vi "Calling_c37_118_LabVIEW_FPGA_test.vi"() -> ()   [LabVIEW 2013]
uses:
  ieeeC37_118.dll
  pmuConnectionData.dll
  <vilib>/rvi/interface/nirviReadWriteControl/nirviReadWriteControl.xnode
  <vilib>/rvi/interface/nirviOpenFPGA/nirviOpenFPGA.xnode
  <vilib>/rvi/interface/nirviCloseFPGA/nirviCloseFPGA.xnode
  FPGA Bitfiles/TestFPGA_FPGATarget_FPGA_R0cnGzbE3PM.lvbitx
  FPGA.vi
  <vilib>/FPGAPlugInAG/cRIO-9081/niLvFpga_Open_cRIO-9081.vi
  <vilib>/rvi/interface/common/dynamic/niFpgaDynamicAddResources.vi
  NiFpgaLv.dll
  <vilib>/Utility/error.llb/Error Cluster From Error Code.vi
  <vilib>/rvi/interface/Simulation/niFpgaSimulationCallBeginRW.vi
  <vilib>/rvi/errors/niLvFpgaAdjustHostInterfaceError.vi
  <vilib>/FPGAPlugInAG/Dynamic/niLvFpga_Close_Dynamic.vi
panel:
  in  "Hold Time":sgl=5000.0
  in  "alpha_POD":sgl=2.0
  in  "alpha_Load":sgl=1.81246
  in  "Scaling_Loadcontrol":sgl=120.0
  in  "Scaling_PhasorPOD":sgl=100.0
  in  "Freq of Osc POD":sgl=0.64
  in  "Freq of Osc Load":sgl=0.64
  out "Loop period monitoring 2":u8
  in  "FPGA Loop  Timer":u8=50
  out "Loop period monitoring":u32
  out "FPGA error":errorcluster
  out "Loop period RT":u8
  out "Samples\nReceived":i32
  in  "Tab Control 4":enum32{"PMUs Data Stream"}(tab)
  out "Frequency":sgl[](array[numeric])
  out "ROCOF":sgl[](array[numeric])
  out "Phasors\n(Magnitude)":sgl[](array[numeric])
  out "Phasors\n(Angle-Degree)":sgl[](array[numeric])
  out "Data Time Stamp":T1
  out "Analogs\n(Value)":sgl[](array[numeric])
  out "Phasors\n(Channel Names)":string[](array[string])
  out "Phasors\n(Types)":string[](array[string])
  out "Phasors\n(PMU Names)":string[](array[string])
  out "Analogs\n(Channel Names)":string[](array[string])
  out "Analogs\n(Types)":string[](array[string])
  out "Analogs\n(PMU Names)":string[](array[string])
  out "Data Error Status":string[](array[string])
  out "PMU Sync Status":string[](array[string])
  out "Data Processed":string[](array[string])
  out "PMU Time Quality":string[](array[string])
  out "PMU Unlocked Time":string[](array[string])
  out "PMU Triggered":string[](array[string])
  out "Trigger Reason":string[](array[string])
  in  "Tab Control 3":enum32{"Connection Data"}(tab)
  in  "IP Address (PMU / PDC)":string="130.237.53.177"
  in  "ID CODE":i32=787
  in  "Port Number":i32=38068
  in  "Tab Control 2":enum32{"PMUs Configuration"}(tab)
  out "Number of\nAnalogs":u16[](array[numeric])
  out "Number of\nDigitals":u16[](array[numeric])
  out "Nominal\nFrequency":sgl[](array[numeric])
  out "Configuration\nCount":u16[](array[numeric])
  out "Number of\nPhasors":u16[](array[numeric])
  out "Station\nName":string[](array[string])
  out "ID Code":u16[](array[numeric])
  in  "Tab Control":enum32{"PDC Configuration"}(tab)
  out "Data Rate:":u16
  out "Number of PMUs:":u16
  out "Configuration Time Stamp":T2
  in  "Shut Down":bool
  out "Error with dll client":errorcluster
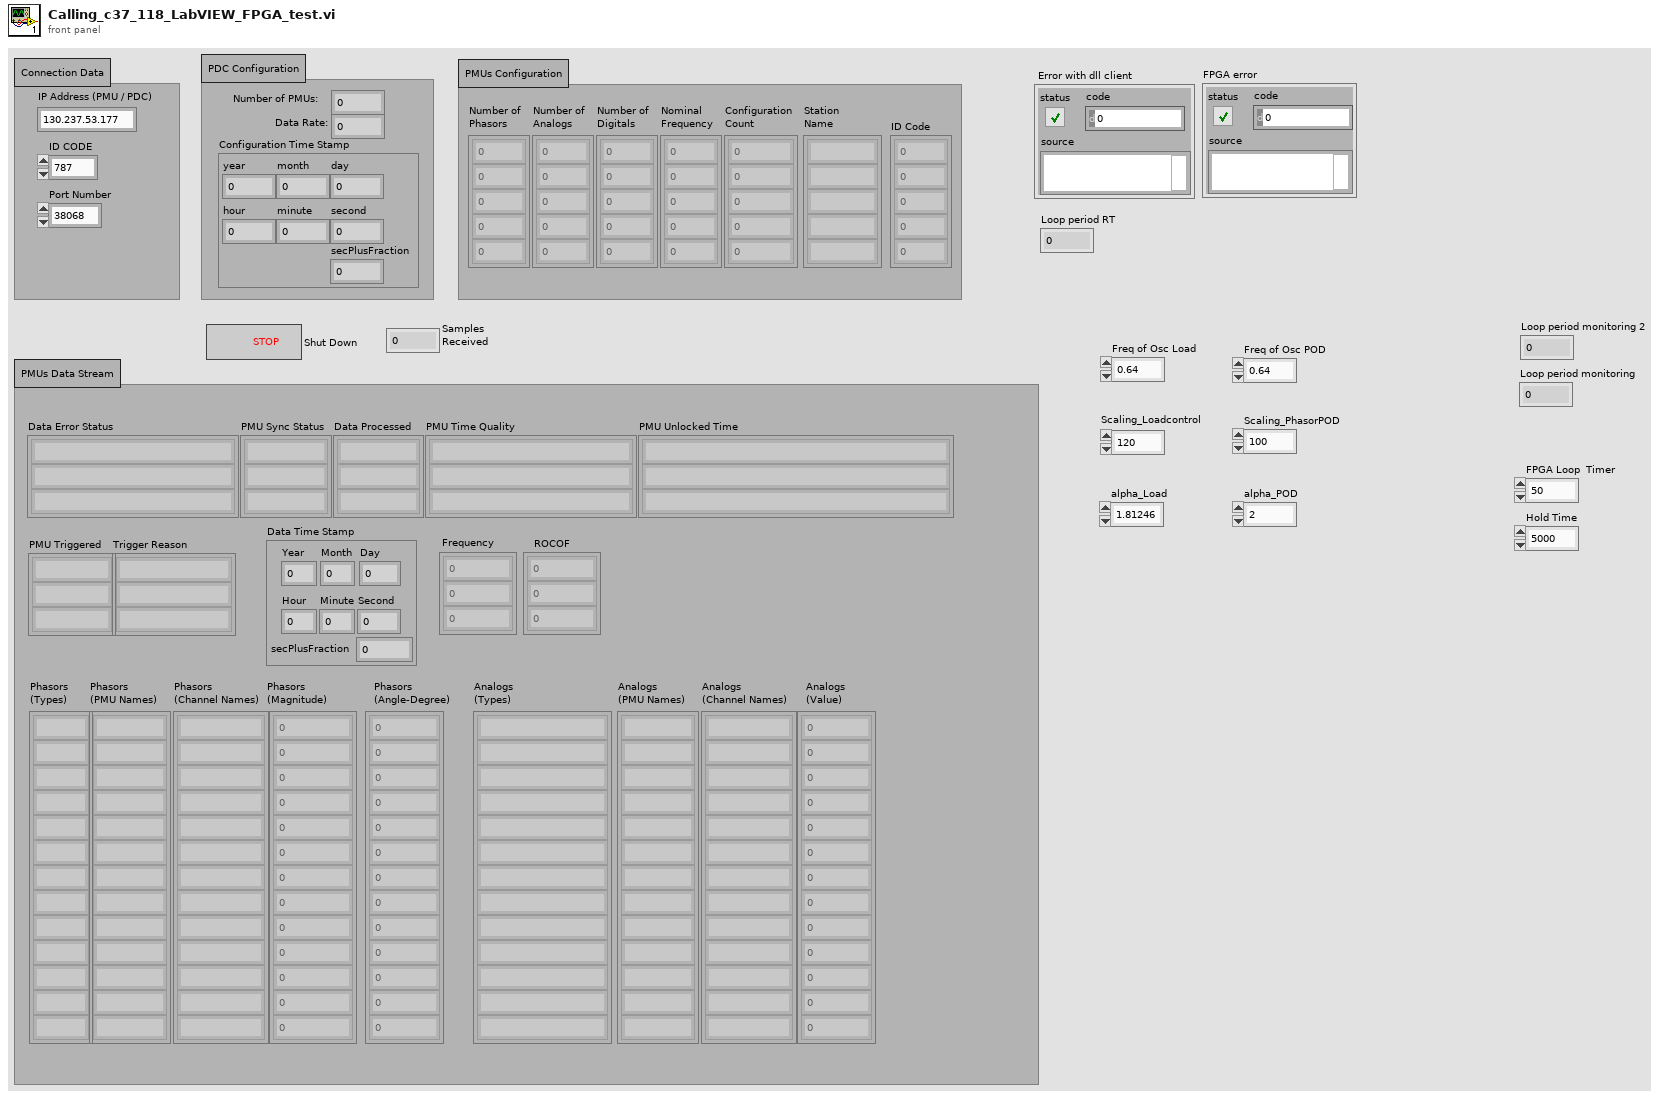
[diagram p1: front panel]
types:
  T1 = cluster{"Year":i32, "Month":i32, "Day":i32, "Hour":i32, "Minute":i32, "Second":i32, "secPlusFraction":sgl}
  T2 = cluster{"year":i32, "month":i32, "day":i32, "hour":i32, "minute":i32, "second":i32, "secPlusFraction":sgl}
  T3 = cluster{"dataError":u8, "dataModified":u8, "pmuIsNOTSync":u8, "pmuIsTriggered":u8, "pmuTimeQuality":u8, "triggerReason":u8, "unlockTime":u8}
  T4 = cluster{"Parameters":cluster{"Ts":sgl, "kappaav":sgl, "kappaph":sgl, "mu":sgl}}
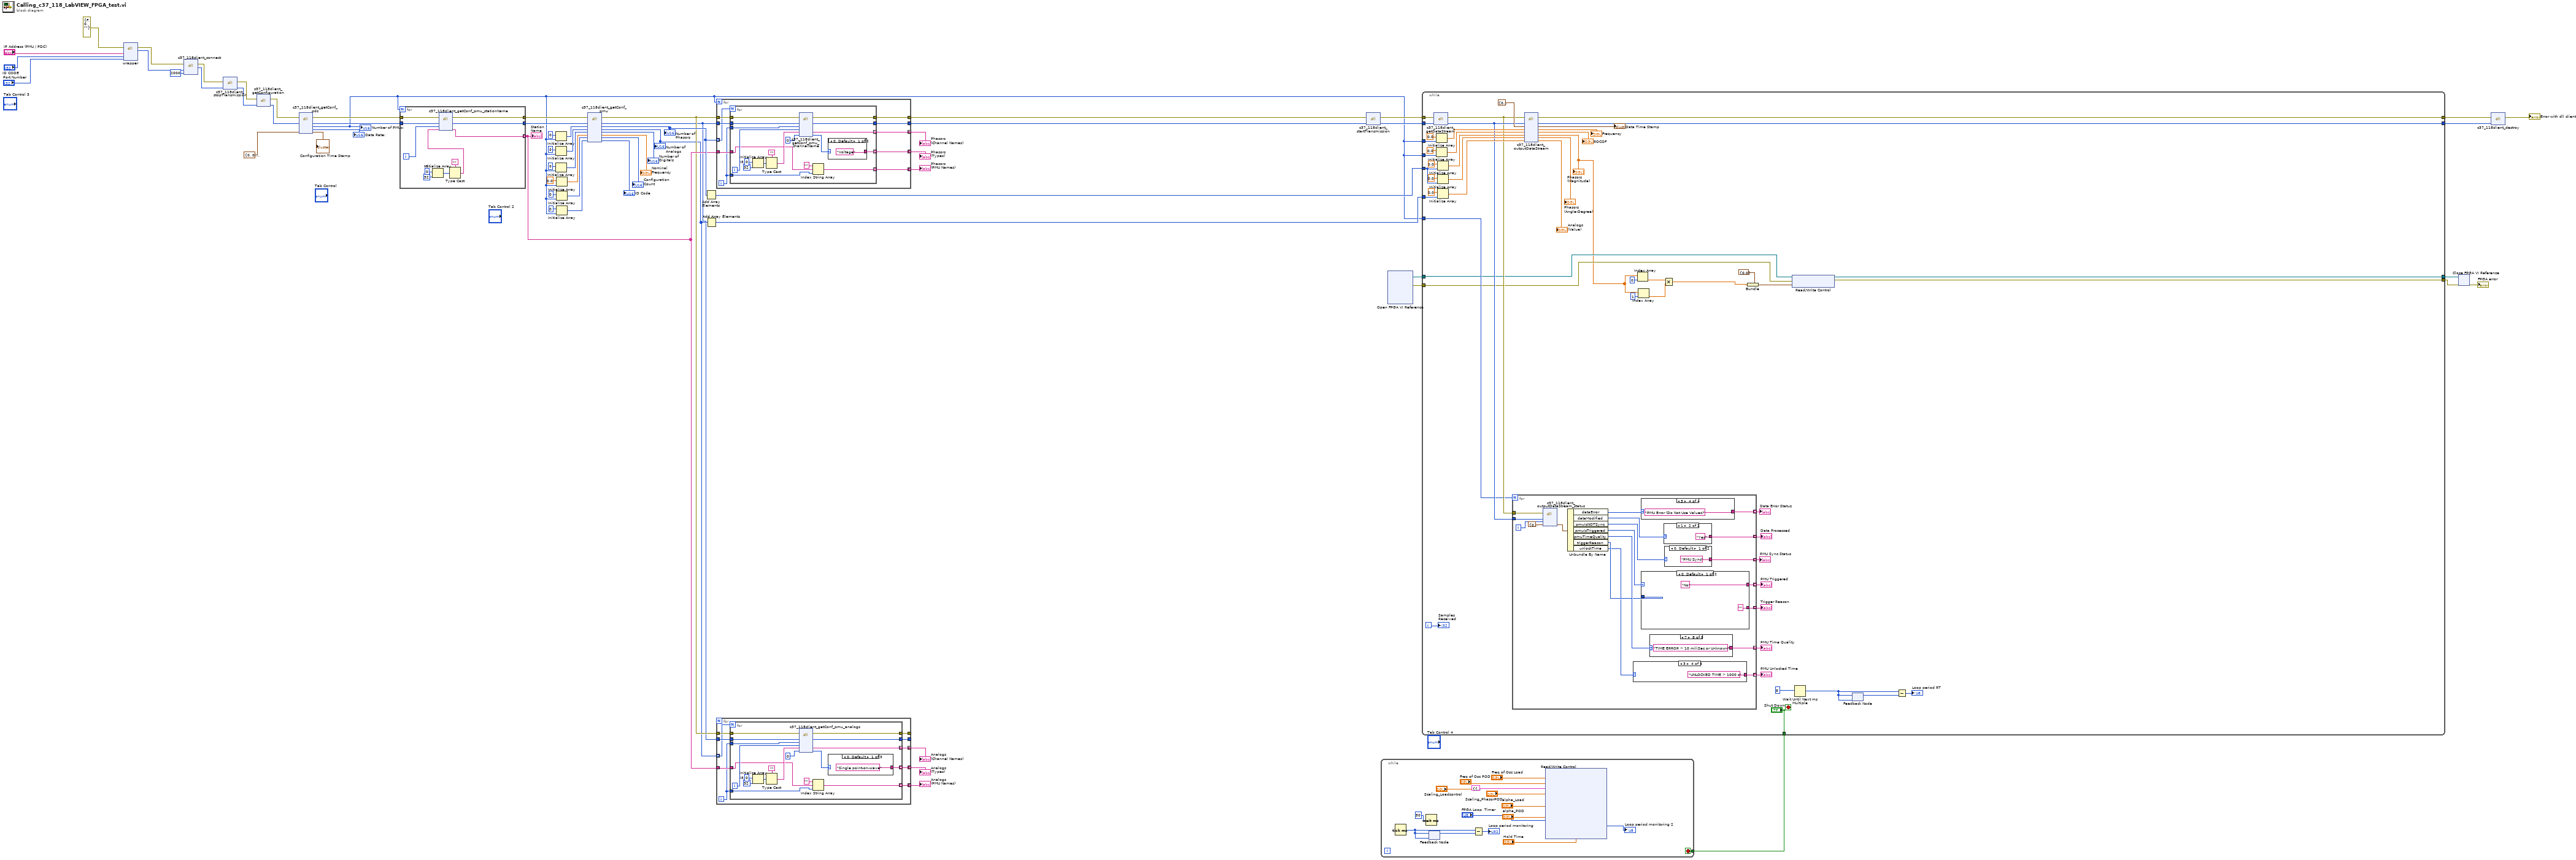
[diagram p0: block diagram]
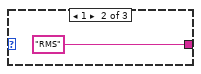
[diagram p2: hidden frame]
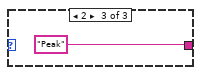
[diagram p3: hidden frame]
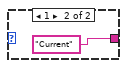
[diagram p4: hidden frame]
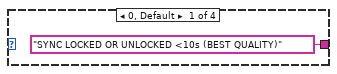
[diagram p5: hidden frame]
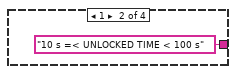
[diagram p6: hidden frame]
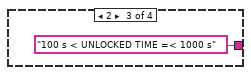
[diagram p7: hidden frame]
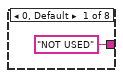
[diagram p8: hidden frame]
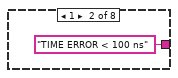
[diagram p9: hidden frame]
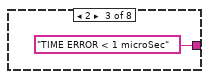
[diagram p10: hidden frame]
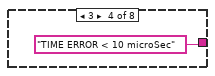
[diagram p11: hidden frame]
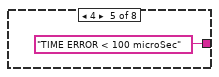
[diagram p12: hidden frame]
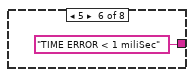
[diagram p13: hidden frame]
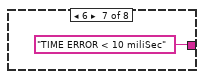
[diagram p14: hidden frame]
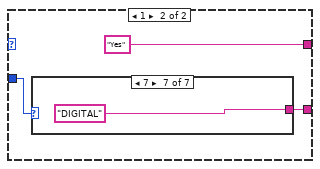
[diagram p15: hidden frame]
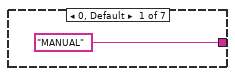
[diagram p16: hidden frame]
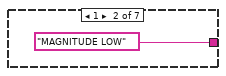
[diagram p17: hidden frame]
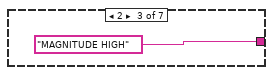
[diagram p18: hidden frame]
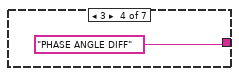
[diagram p19: hidden frame]
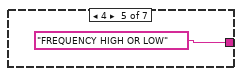
[diagram p20: hidden frame]
diagram:
  n1 = dll-call lib="pmuConnectionData.*" fn="wrapper"(error in=errorcluster {"status"=FALSE, "code"=0, "source"=""} ("error in (no error)"), "ipAddress_PmuServer"="IP Address (PMU / PDC)", "pmuPortNumber"="ID CODE", "pmuIdCode"="Port Number") -> (error out=w54:errorcluster, "PMUConnectionData"=w63:i64)  [unwired: 5 in, 1 out]
  n2 = dll-call lib="ieeeC37_118.*" fn="c37_118client_connect"(error in=w54, "parameters"=w63, "timeoutInMs"=u32 2000) -> (error out=w53:errorcluster, "c37_118Object"=w61:i64)  [unwired: 4 in, 1 out]
  n3 = dll-call lib="ieeeC37_118.dll" fn="c37_118client_stopTransmission"(error in=w53, "self"=w61) -> (error out=w52:errorcluster, "self"=w60:i64)  [unwired: 3 in, 1 out]
  n4 = dll-call lib="ieeeC37_118.dll" fn="c37_118client_getConfiguration"(error in=w52, "self"=w60) -> (error out=w51:errorcluster, "self"=w57:i64)  [unwired: 3 in, 1 out]
  n5 = dll-call lib="ieeeC37_118.dll" fn="c37_118client_getConf_pdc"(error in=w51, "self"=w57, "timestamp"=T2 {"year"=0, "month"=0, "day"=0, "hour"=0, "minute"=0, "second"=0, "secPlusFraction"=0.0}) -> (error out=w28:errorcluster, "self"=w26:i64, "num_pmu"=w7:u16, "data_rate"=→"Data Rate:":u16, "timestamp"=→"Configuration Time Stamp":T2)  [unwired: 5 in, 1 out]
  "Number of PMUs:" <- w7
  n6 = for {
    N: w7 -> [_]
    tunnel: w28 -> [w74]
    tunnel: [w73] -> w27
    tunnel: w26 -> [w72]
    tunnel: [w71] -> w25
    tunnel: [w70] -> w11 mode=indexing
    i -> [w64]
    w69 = i8 0  # I8
    n7 = Initialize Array(w69, 32 ("dimension size")) -> (w68:i8[])
    n8 = Type Cast(type="", x=w68) -> (*(type *) &x=w66:string)
    n9 = dll-call lib="ieeeC37_118.dll" fn="c37_118client_getConf_pmu_stationName"(error in=w74, "self"=w72, "pmuNumber"=w64, "stationName"=w66) -> (error out=w73:errorcluster, "self"=w71:i64, "stationName"=w70:string)  [unwired: 4 in, 1 out]
  }
  "Station\nName" <- w11
  n10 = Initialize Array(u16 0 ("element"), w7) -> (w44:u16[])
  n11 = Initialize Array(u16 0 ("element"), w7) -> (w41:u16[])
  n12 = Initialize Array(u16 0 ("element"), w7) -> (w37:u16[])
  n13 = Initialize Array(sgl 0.0 ("element"), w7) -> (w36:sgl[])
  n14 = Initialize Array(u16 0 ("element"), w7) -> (w35:u16[])
  n15 = Initialize Array(u16 0 ("element"), w7) -> (w18:u16[])
  n16 = dll-call lib="ieeeC37_118.dll" fn="c37_118client_getConf_pmu"(error in=w27, "self"=w25, "numPhasors"=w44, "numAnalog"=w41, "numdigital"=w37, "freqNom"=w36, "configCount"=w35, "idCode"=w18) -> (error out=w10:errorcluster, "self"=w8:i64, "numPhasors"=w22:u16[], "numAnalog"=w9:u16[], "numdigital"=→"Number of\nDigitals":u16[], "freqNom"=→"Nominal\nFrequency":sgl[], "configCount"=→"Configuration\nCount":u16[], "idCode"=→"ID Code":u16[])  [unwired: 3 in, 1 out]
  "Number of\nAnalogs" <- w9
  "Number of\nPhasors" <- w22
  n17 = Add Array Elements(numeric array=w22) -> (sum=w24:u16)
  n18 = Add Array Elements(numeric array=w9) -> (sum=w29:u16)
  n19 = for {
    N: w7 -> [_]
    tunnel: w10 -> [w83]
    tunnel: [w82] -> w12
    tunnel: w8 -> [w84]
    tunnel: [w81] -> w13
    tunnel: [w80] -> w23 mode=concatenating
    tunnel: w22 -> [w79] mode=indexing
    tunnel: [w78] -> w21 mode=concatenating
    tunnel: w11 -> [w77]
    tunnel: [w75] -> w20 mode=concatenating
    i -> [w76]
    n20 = for {
      N: w79 -> [_]
      tunnel: w76 -> [w97]
      tunnel: w84 -> [w96]
      tunnel: w83 -> [w95]
      tunnel: [w94] -> w82
      tunnel: [w93] -> w81
      tunnel: [w92] -> w80 mode=indexing
      tunnel: [w89] -> w78 mode=indexing
      tunnel: w77 -> [w87]
      tunnel: w76 -> [w88]
      tunnel: [w85] -> w75 mode=indexing
      i -> [w98]
      w103 = i8 0  # I8
      n21 = Initialize Array(w103, 32 ("dimension size")) -> (w102:i8[])
      n22 = Type Cast(type="", x=w102) -> (*(type *) &x=w99:string)
      n23 = dll-call lib="ieeeC37_118.dll" fn="c37_118client_getConf_pmu_channelName"(error in=w95, "self"=w96, "pmuNumber"=w97, "phasor"=w98, "channelName"=w99, "phasorType"=0) -> (error out=w94:errorcluster, "self"=w93:i64, "channelName"=w92:string, "phasorType"=w90:i32)  [unwired: 5 in, 1 out]
      n24 = Index String Array(1:w88, 2:w87, 3:"" ("string (\"\")")) -> (0:w85:string)
      n25 = case shown="0, Default" w90 {
        tunnel: ["Voltage" "Current"] -> w89
        frame 0, Default {
        }
        frame 1 {
        }
      }
    }
  }
  "Phasors\n(Channel Names)" <- w23
  "Phasors\n(Types)" <- w21
  "Phasors\n(PMU Names)" <- w20
  n26 = for {
    tunnel: w10 -> [w114]
    tunnel: [w113] -> _
    tunnel: w8 -> [w115]
    tunnel: [w112] -> _
    tunnel: [w111] -> w16 mode=concatenating
    tunnel: w9 -> [w110] mode=indexing
    tunnel: [w109] -> w15 mode=concatenating
    tunnel: w11 -> [w108]
    tunnel: [w106] -> w14 mode=concatenating
    i -> [w107]
    n27 = for {
      N: w110 -> [_]
      tunnel: w107 -> [w128]
      tunnel: w115 -> [w127]
      tunnel: w114 -> [w126]
      tunnel: [w125] -> w113
      tunnel: [w124] -> w112
      tunnel: [w123] -> w111 mode=indexing
      tunnel: [w120] -> w109 mode=indexing
      tunnel: w108 -> [w118]
      tunnel: w107 -> [w119]
      tunnel: [w116] -> w106 mode=indexing
      i -> [w129]
      w134 = i8 0  # I8
      n28 = Initialize Array(w134, 32 ("dimension size")) -> (w133:i8[])
      n29 = Type Cast(type="", x=w133) -> (*(type *) &x=w130:string)
      n30 = dll-call lib="ieeeC37_118.dll" fn="c37_118client_getConf_pmu_analogs"(error in=w126, "self"=w127, "pmuNumber"=w128, "analog"=w129, "channelName"=w130, "analogType"=0 ("phasorType")) -> (error out=w125:errorcluster, "self"=w124:i64, "channelName"=w123:string, "analogType"=w121:i32)  [unwired: 5 in, 1 out]
      n31 = Index String Array(1:w119, 2:w118, 3:"" ("string (\"\")")) -> (0:w116:string)
      n32 = case shown="0, Default" w121 {
        tunnel: ["Single point-on-wave" "RMS" "Peak"] -> w120
        frame 0, Default {
        }
        frame 1 {
        }
        frame 2 {
        }
      }
    }
  }
  "Analogs\n(Channel Names)" <- w16
  "Analogs\n(Types)" <- w15
  "Analogs\n(PMU Names)" <- w14
  n33 = dll-call lib="ieeeC37_118.dll" fn="c37_118client_startTransmission"(error in=w12, "self"=w13) -> (error out=w50:errorcluster, "self"=w59:i64)  [unwired: 3 in, 1 out]
  n34 = xnode "Open FPGA VI Reference"() -> ("FPGA VI Reference Out"=w6:refnum<k20>, "error out"=w5:errorcluster)  [unwired: 2 in]
  n35 = while {
    tunnel: w59 -> [w189]
    tunnel: [w186] -> w58
    tunnel: w50 -> [w188]
    tunnel: [w187] -> w49
    tunnel: w7 -> [w184]
    tunnel: w7 -> [w181]
    tunnel: w24 -> [w175]
    tunnel: w29 -> [w168]
    tunnel: w7 -> [w164]
    tunnel: w6 -> [w149]
    tunnel: w5 -> [w150]
    tunnel: [w148] -> w4
    tunnel: [w147] -> w3
    tunnel: ["Shut Down"] -> w1
    i -> [w170]
    stop <- "Shut Down" stop-if-true
    n36 = dll-call lib="ieeeC37_118.dll" fn="c37_118client_getDataStream"(error in=w188, "self"=w189) -> (error out=w165:errorcluster, "self"=w166:i64)  [unwired: 3 in, 1 out]
    n37 = Initialize Array(sgl 0.0 ("element"), w184) -> (w183:sgl[])
    n38 = Initialize Array(sgl 0.0 ("element"), w181) -> (w180:sgl[])
    n39 = Initialize Array(sgl 0.0 ("element"), w175) -> (w174:sgl[])
    n40 = Initialize Array(sgl 0.0 ("element"), w175) -> (w173:sgl[])
    n41 = Initialize Array(sgl 0.0 ("element"), w168) -> (w167:sgl[])
    n42 = for {
      N: w164 -> [_]
      tunnel: w166 -> [w208]
      tunnel: w165 -> [w207]
      tunnel: [w204] -> w163 mode=indexing
      tunnel: [w201] -> w162 mode=indexing
      tunnel: [w198] -> w161 mode=indexing
      tunnel: [w196] -> w160 mode=indexing
      tunnel: [w195] -> w159 mode=indexing
      tunnel: [w192] -> w158 mode=indexing
      tunnel: [w190] -> w157 mode=indexing
      i -> [w206]
      n43 = dll-call lib="ieeeC37_118.dll" fn="c37_118client_outputDataStream_status"(error in=w207, "self"=w208, "pmuNumber"=w206, "status"=T3 {"dataError"=0, "dataModified"=0, "pmuIsNOTSync"=0, "pmuIsTriggered"=0, "pmuTimeQuality"=0, "triggerReason"=0, "unlockTime"=0}) -> ("status"=w203:T3)  [unwired: 5 in, 2 out]
      n44 = Unbundle By Name(w203) -> ("dataError"=w200:u8, "dataModified"=w199:u8, "pmuIsNOTSync"=w202:u8, "pmuIsTriggered"=w197:u8, "pmuTimeQuality"=w194:u8, "triggerReason"=w193:u8, "unlockTime"=w191:u8)
      n45 = case shown="3" w191 {
        tunnel: ["SYNC LOCKED OR UNLOCKED <10s (BEST QUALITY)" "10 s =< UNLOCKED TIME < 100 s" "100 s < UNLOCKED TIME =< 1000 s" "UNLOCKED TIME > 1000 s"] -> w190
        frame 0, Default {
        }
        frame 1 {
        }
        frame 2 {
        }
        frame 3 {
        }
      }
      n46 = case shown="3" w200 {
        tunnel: ["Good Measurment Data (No Errors)" "PMU Error, No Information About Data" "PMU In Test Mode (Do Not Use Values)" "PMU Error (Do Not Use Values)"] -> w204
        frame 0, Default {
        }
        frame 1 {
        }
        frame 2 {
        }
        frame 3 {
        }
      }
      n47 = case shown="0, Default" w197 {
        tunnel: ["No" "Yes"] -> w196
        tunnel: w193 -> [_ w224]
        tunnel: ["" w223] -> w192
        frame 0, Default {
        }
        frame 1 {
          n48 = case shown="7" w224 {
            tunnel: ["MANUAL" "MAGNITUDE LOW" "MAGNITUDE HIGH" "PHASE ANGLE DIFF" "FREQUENCY HIGH OR LOW" "df/dt HIGH" "DIGITAL"] -> w223
            frame 0, Default {
            }
            frame 1 {
            }
            frame 2 {
            }
            frame 3 {
            }
            frame 4 {
            }
            frame 5 {
            }
            frame 7 {
            }
          }
        }
      }
      n49 = case shown="7" w194 {
        tunnel: ["NOT USED" "TIME ERROR < 100 ns" "TIME ERROR < 1 microSec" "TIME ERROR < 10 microSec" "TIME ERROR < 100 microSec" "TIME ERROR < 1 miliSec" "TIME ERROR < 10 miliSec" "TIME ERROR > 10 miliSec or Unknown"] -> w195
        frame 0, Default {
        }
        frame 1 {
        }
        frame 2 {
        }
        frame 3 {
        }
        frame 4 {
        }
        frame 5 {
        }
        frame 6 {
        }
        frame 7 {
        }
      }
      n50 = case shown="1" w199 {
        tunnel: ["No" "Yes"] -> w198
        frame 0, Default {
        }
        frame 1 {
        }
      }
      n51 = case shown="0, Default" w202 {
        tunnel: ["PMU Sync" "PMU Not Sync"] -> w201
        frame 0, Default {
        }
        frame 1 {
        }
      }
    }
    "Data Error Status" <- w163
    "PMU Sync Status" <- w162
    "Data Processed" <- w161
    "PMU Triggered" <- w160
    "PMU Time Quality" <- w159
    "Trigger Reason" <- w158
    "PMU Unlocked Time" <- w157
    n52 = dll-call lib="ieeeC37_118.dll" fn="c37_118client_outputDataStream"(error in=w165, "self"=w166, "timestamp"=T2 {"year"=0, "month"=0, "day"=0, "hour"=0, "minute"=0, "second"=0, "secPlusFraction"=0.0}, "freqBuffer"=w183, "rocofBuffer"=w180, "phasorsMagBuffer"=w174, "phasorsAngBuffer"=w173, "analogBuffer"=w167) -> (error out=w187:errorcluster, "self"=w186:i64, "timestamp"=→"Data Time Stamp":T2, "freqBuffer"=→"Frequency":sgl[], "rocofBuffer"=→"ROCOF":sgl[], "phasorsMagBuffer"=w139:sgl[], "phasorsAngBuffer"=→"Phasors\n(Angle-Degree)":sgl[], "analogBuffer"=→"Analogs\n(Value)":sgl[])  [unwired: 3 in, 1 out]
    "Phasors\n(Magnitude)" <- w139
    n53 = Index Array(array=w139, index=0) -> (element=w143:sgl)
    n54 = Index Array(array=w139, index=1) -> (element=w142:sgl)
    n55 = Multiply(x=w143, y=w142) -> (x*y=w141:sgl)
    n56 = Bundle(cluster=cluster{sgl} {0.0}, w141) -> (w146:cluster{sgl})
    n57 = xnode "Read/Write Control"("FPGA VI Reference In"=w149, "error in"=w150, "PMU measurments"=w146) -> ("FPGA VI Reference Out"=w148:refnum<k20>, "error out"=w147:errorcluster)
    n58 = Wait Until Next ms Multiple(millisecond multiple=u32 5) -> (millisecond timer value=w152:u32)
    n59 = feedback #1(w152) -> (w154:u32)
    n60 = feedback-in #1(w152) -> ()
    n61 = Subtract(x=w152, y=w154) -> (x-y=→"Loop period RT":u32)
    "Samples\nReceived" <- w170
  }
  n62 = while {
    tunnel: w1 -> [w241]
    stop <- w241 stop-if-true
    n63 = Tick Count (ms)() -> (millisecond timer value=w254:u32)
    n64 = Wait (ms)(milliseconds to wait=u32 50) -> ()  [unwired: 1 out]
    n65 = feedback #2(w254) -> (w253:u32)
    n66 = feedback-in #2(w254) -> ()
    n67 = Subtract(x=w254, y=w253) -> (x-y=→"Loop period monitoring":u32)
    n68 = xnode "Read/Write Control"("Freq of Osc Load"="Freq of Osc Load", "Freq of Osc POD"="Freq of Osc POD", "Frequency Estimator Settings"=T4 {"Parameters"={"Ts"=5e-05, "kappaav"=0.625, "kappaph"=0.5762, "mu"=0.7086}}, "Scaling_PhasorPOD"="Scaling_PhasorPOD", "Scaling_Loadcontrol"="Scaling_Loadcontrol", "alpha_Load"="alpha_Load", "alpha_POD"="alpha_POD", "FPGA Loop  Timer"="FPGA Loop  Timer", "Hold Time"="Hold Time") -> ("Loop period monitoring"=→"Loop period monitoring 2":u8)  [unwired: 2 in, 4 out]
  }
  n69 = xnode "Close FPGA VI Reference"("FPGA VI Reference In"=w4, "error in"=w3) -> ("error out"=→"FPGA error":errorcluster)
  n70 = dll-call lib="ieeeC37_118.dll" fn="c37_118client_destroy"(error in=w49, "self"=w58) -> (error out=→"Error with dll client":errorcluster)  [unwired: 4 in, 1 out]
